vi "InitShooter.vi"   [LabVIEW 2019]
doc: "This VI initializes devices related directly to the shooter and turret subsystems."
uses:
  refnums.vi
  <vilib>/Rock Robotics/WPI/ThirdParty/REV Robotics/SPARK MAX/Typedef/Spark MAX Idle Mode.ctl
  <vilib>/Rock Robotics/WPI/Solenoid/WPI_SolenoidChannel.ctl
  <vilib>/Rock Robotics/WPI/Solenoid/WPI_SolenoidOpenDouble.vi
  <vilib>/Rock Robotics/SystemInterfaces/DIO/FPGA_DIOPWMChannel.ctl
types:
  T1 = typedef "FPGA_DIOPWMChannel.ctl" = enum8{"PWM 0", "PWM 1", "PWM 2", "PWM 3", "PWM 4", "PWM 5", "PWM 6", "PWM 7", "PWM 8", "PWM 9", "PWM MXP 0", "PWM MXP 1", "PWM MXP 2", "PWM MXP 3", "PWM MXP 4", "PWM MXP 5", "PWM MXP 6", "PWM MXP 7", "PWM MXP 8", "PWM MXP 9", "Invalid"}
  T2 = typedef "WPI_SolenoidChannel.ctl" = enum8{"Solenoid 0", "Solenoid 1", "Solenoid 2", "Solenoid 3", "Solenoid 4", "Solenoid 5", "Solenoid 6", "Solenoid 7", "Invalid"}
  T3 = typedef "Spark MAX Idle Mode.ctl" = enum16{"Coast", "Brake"}
  T4 = typedef "WPI_MotorControlDeviceRef.ctl" = cluster{"DeviceStatus":errorcluster, "Type":T5, "PWM":cluster{"PWM Channel":T1, "DeadBand":T6}, "CAN":cluster{"Device Number":u8, "SetOutput VI Ref":variant, "GetOutput VI Ref":variant, "Enable VI Ref":variant, "Disable VI Ref":variant, "Data":variant}, "Invert":bool, "DIO PWM":cluster{"PWM \"Enable\" Channel":T1, "DIOChannel":T7, "PWM Rate":dbl}}
  T5 = typedef "WPI_MotorControlType.ctl" = enum16{"PWM", "CAN", "DIO PWM"}
  T6 = typedef "WPI_PWMDeadband.ctl" = cluster{"Name":string, "maxPositivePwm":i32, "minPositivePwm":i32, "centerPwm":i32, "maxNegativePwm":i32, "minNegativePwm":i32, "angularRange":u16}
  T7 = typedef "FPGA_DIOChannel.ctl" = enum8{"DIO 0", "DIO 1", "DIO 2", "DIO 3", "DIO 4", "DIO 5", "DIO 6", "DIO 7", "DIO 8", "DIO 9", "DIO MXP 0", "DIO MXP 1", "DIO MXP 2", "DIO MXP 3", "DIO MXP 4", "DIO MXP 5", "DIO MXP 6", "DIO MXP 7", "DIO MXP 8", "DIO MXP 9", "DIO MXP 10", "DIO MXP 11", "DIO MXP 12", "DIO MXP 13", "DIO MXP 14", "DIO MXP 15", "SPI Port CS1", "SPI Port CS2", "SPI Port CS3", "SPI Port MISO", "SPI Port MOSI", "Invalid"}
  T8 = typedef "WPI_ServoDeviceRef.ctl" = cluster{"DeviceStatus":errorcluster, "PWM Channel":T1, "DeadBand":T6}
  T9 = typedef "WPI_SolenoidDevRef.ctl" = cluster{"DevStatus":errorcluster, "Pneumatics Control Module":u8, "Forward Solenoid Channel":T2, "Reverse Solenoid Channel":T2}
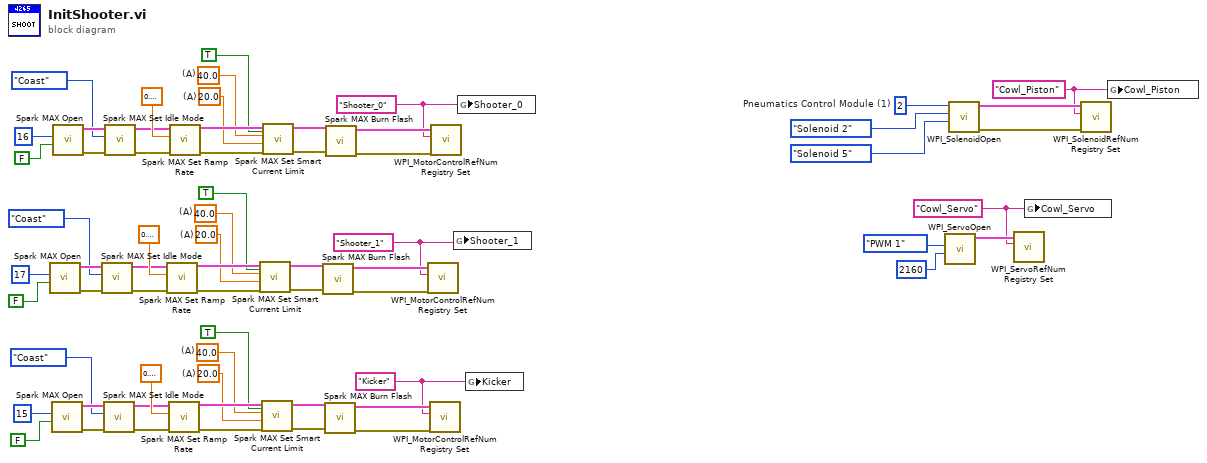
[diagram p0: block diagram]
diagram:
  w3 = "Cowl_Servo" ("refnum name")
  w5 = "Cowl_Piston" ("refnum name")
  w10 = u8 2  # Pneumatics Control Module (1)
  w18 = 40.0  # (A)
  w17 = 20.0  # (A)
  w14 = "Kicker" ("refnum name")
  w39 = 40.0  # (A)
  w38 = 20.0  # (A)
  w34 = "Shooter_1" ("refnum name")
  w53 = 40.0  # (A)
  w52 = 20.0  # (A)
  w35 = "Shooter_0" ("refnum name")
  n1 = call <vilib>:"Spark MAX Open.vi"("Invert"=FALSE, "Device Number"=u8 17 ("Drive 1R")) -> ("error out"=w46:errorcluster, "MotorControlDeviceRef"=w49:T4)  [unwired: 8 in]
  n2 = call <vilib>:"Spark MAX Open.vi"("Invert"=FALSE, "Device Number"=u8 15 ("Drive 1R")) -> ("error out"=w25:errorcluster, "MotorControlDeviceRef"=w28:T4)  [unwired: 8 in]
  n3 = call <vilib>:"Spark MAX Open.vi"("Invert"=FALSE, "Device Number"=u8 16 ("Drive 1R")) -> ("error out"=w60:errorcluster, "MotorControlDeviceRef"=w63:T4)  [unwired: 8 in]
  n4 = call <vilib>:"Spark MAX Set Idle Mode.vi"("error in (no error)"=w46, "Idle Mode"=Spark_MAX_Idle_Mode."Coast", "MotorControlDeviceRef in"=w49) -> ("error out"=w32:errorcluster, "MotorControlDeviceRef out"=w33:T4)  [unwired: 7 in]
  n5 = call <vilib>:"Spark MAX Set Idle Mode.vi"("error in (no error)"=w25, "Idle Mode"=Spark_MAX_Idle_Mode."Coast", "MotorControlDeviceRef in"=w28) -> ("error out"=w12:errorcluster, "MotorControlDeviceRef out"=w13:T4)  [unwired: 7 in]
  n6 = call <vilib>:"Spark MAX Set Idle Mode.vi"("error in (no error)"=w60, "Idle Mode"=Spark_MAX_Idle_Mode."Coast", "MotorControlDeviceRef in"=w63) -> ("error out"=w30:errorcluster, "MotorControlDeviceRef out"=w31:T4)  [unwired: 7 in]
  n7 = call <vilib>:"Spark MAX Set Ramp Rate.vi"("error in (no error)"=w32, "Seconds from neutral to full (0)"=sgl 0.2, "MotorControlDeviceRef in"=w33) -> ("error out"=w43:errorcluster, "MotorControlDeviceRef"=w40:T4)  [unwired: 7 in]
  n8 = call <vilib>:"Spark MAX Set Ramp Rate.vi"("error in (no error)"=w12, "Seconds from neutral to full (0)"=sgl 0.2, "MotorControlDeviceRef in"=w13) -> ("error out"=w22:errorcluster, "MotorControlDeviceRef"=w19:T4)  [unwired: 7 in]
  n9 = call <vilib>:"Spark MAX Set Ramp Rate.vi"("error in (no error)"=w30, "Seconds from neutral to full (0)"=sgl 0.2, "MotorControlDeviceRef in"=w31) -> ("error out"=w57:errorcluster, "MotorControlDeviceRef"=w54:T4)  [unwired: 7 in]
  n10 = call <vilib>:"Spark MAX Set Smart Current Limit.vi"("Linearized Limit Enabled (F)"=TRUE, "error in (no error)"=w43, "Free Speed Current Limit (20A)"=w38, "Primay Current Limit (80A)"=w39, "MotorControlDeviceRef in"=w40) -> ("error out"=w42:errorcluster, "MotorControlDeviceRef out"=w41:T4)  [unwired: 5 in]
  n11 = call <vilib>:"Spark MAX Set Smart Current Limit.vi"("Linearized Limit Enabled (F)"=TRUE, "error in (no error)"=w22, "Free Speed Current Limit (20A)"=w17, "Primay Current Limit (80A)"=w18, "MotorControlDeviceRef in"=w19) -> ("error out"=w21:errorcluster, "MotorControlDeviceRef out"=w20:T4)  [unwired: 5 in]
  n12 = call <vilib>:"Spark MAX Set Smart Current Limit.vi"("Linearized Limit Enabled (F)"=TRUE, "error in (no error)"=w57, "Free Speed Current Limit (20A)"=w52, "Primay Current Limit (80A)"=w53, "MotorControlDeviceRef in"=w54) -> ("error out"=w56:errorcluster, "MotorControlDeviceRef out"=w55:T4)  [unwired: 5 in]
  n13 = call <vilib>:"Spark MAX Burn Flash.vi"("error in"=w42, "MotorControlDeviceRef"=w41) -> ("error out"=w44:errorcluster, "MotorControlDeviceRef"=w45:T4)  [unwired: 8 in]
  n14 = call <vilib>:"Spark MAX Burn Flash.vi"("error in"=w21, "MotorControlDeviceRef"=w20) -> ("error out"=w23:errorcluster, "MotorControlDeviceRef"=w24:T4)  [unwired: 8 in]
  n15 = call <vilib>:"Spark MAX Burn Flash.vi"("error in"=w56, "MotorControlDeviceRef"=w55) -> ("error out"=w58:errorcluster, "MotorControlDeviceRef"=w59:T4)  [unwired: 8 in]
  n16 = call <vilib>:"WPI_MotorControlRefNum Registry Set.vi"("error in (no error)"=w44, "refnum name"=w34, "MotorControlDevRef"=w45) -> ()  [unwired: 7 in, 2 out]
  n17 = call <vilib>:"WPI_MotorControlRefNum Registry Set.vi"("error in (no error)"=w23, "refnum name"=w14, "MotorControlDevRef"=w24) -> ()  [unwired: 7 in, 2 out]
  n18 = call <vilib>:"WPI_MotorControlRefNum Registry Set.vi"("error in (no error)"=w58, "refnum name"=w35, "MotorControlDevRef"=w59) -> ()  [unwired: 7 in, 2 out]
  n19 = global write "refnums.vi" "Shooter_1"(w34) -> ()
  n20 = global write "refnums.vi" "Shooter_0"(w35) -> ()
  n21 = global write "refnums.vi" "Kicker"(w14) -> ()
  n22 = call <vilib>:"WPI_ServoOpen.vi"("Angular Range"=u16 2160, "PWM Channel"=FPGA_DIOPWMChannel."PWM 1") -> ("ServoDeviceRef"=w4:T8)  [unwired: 8 in, 1 out]
  n23 = call-poly <vilib>:"WPI_SolenoidOpen.vi"("Reverse Solenoid Channel"=WPI_SolenoidChannel."Solenoid 5", "Forward Solenoid Channel"=WPI_SolenoidChannel."Solenoid 2", "Pneumatics Control Module (0)"=w10) -> ("error out"=w6:errorcluster, "SolenoidDevRef"=w7:T9)  [unwired: 7 in]
  n24 = call <vilib>:"WPI_ServoRefNum Registry Set.vi"("refnum name"=w3, "ServoDeviceRef"=w4) -> ()  [unwired: 8 in, 2 out]
  n25 = global write "refnums.vi" "Cowl_Servo"(w3) -> ()
  n26 = call <vilib>:"WPI_SolenoidRefNum Registry Set.vi"("error in (no error)"=w6, "refnum name"=w5, "SolenoidDevRef"=w7) -> ()  [unwired: 7 in, 2 out]
  n27 = global write "refnums.vi" "Cowl_Piston"(w5) -> ()
